vi "set output trigger source.vi"(8 "error in (no error)":errorcluster, 10 "Output trigger connector":T1=enum."3", 11 "DAQOrcaFlash in":refnum<class "DAQOrcaFlash.lvclass">) -> (0 "error out":errorcluster, 3 "DAQOrcaFlash out":refnum<class "DAQOrcaFlash.lvclass">)   [LabVIEW 2012, in "DAQOrcaFlash.lvclass"]
uses:
  DAQOrcaFlash.lvclass
  connector.ctl
  DAQOrcaFlash.lvclass/DAQOrcaFlash.ctl
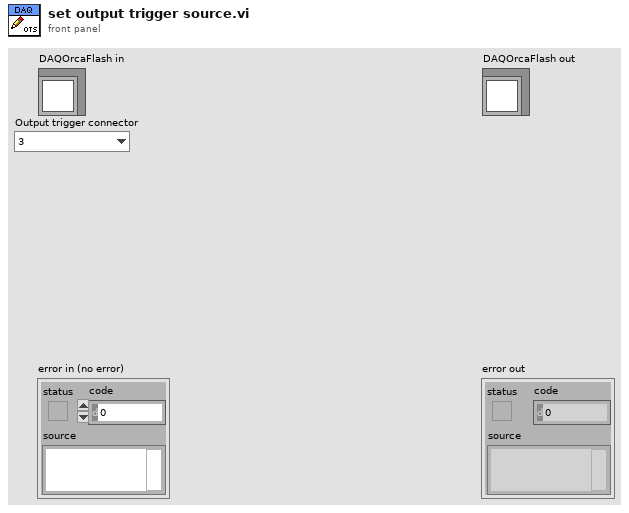
[diagram p1: front panel]
types:
  T1 = typedef "DAQOrcaFlash.lvclass/connector.ctl" = enum32{"1", "2", "3"}
  T2 = typedef "DAQOrcaFlash.lvclass/output trigger source.ctl" = sgl
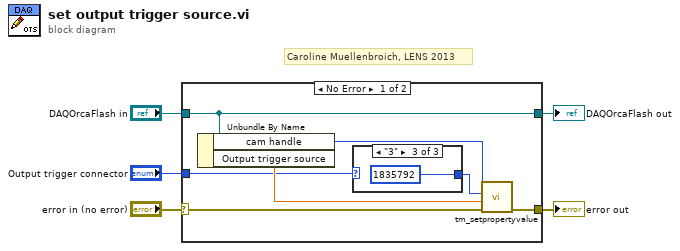
[diagram p0: block diagram]
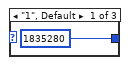
[diagram p2: hidden frame]
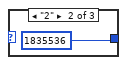
[diagram p3: hidden frame]
diagram:
  # "Caroline Muellenbroich, LENS 2013"
  n1 = case shown="No Error" "error in (no error)" {
    selector: "error in (no error)" -> [w11 w17]
    tunnel: [w10 w17] -> w4
    tunnel: [w12 w16] -> w2
    tunnel: "DAQOrcaFlash in" -> [w12 w16]
    tunnel: "Output trigger connector" -> [w6 _]
    frame No Error {
      n2 = Unbundle By Name(w12) -> ("cam handle"=w8:u32, "Output trigger source"=w9:T2)
      n3 = case shown="\"3\"" w6 {
        tunnel: [u32 1835280 ("Property ID") u32 1835536 ("Property ID") u32 1835792 ("Property ID")] -> w7
        frame "1", Default {
        }
        frame "2" {
        }
        frame "3" {
        }
      }
      n4 = call <userlib>:"tm_setpropertyvalue.vi"("error in (no error)"=w11, "Value in"=w9, "Property ID"=w7, "Handle in"=w8) -> ("error out"=w10:errorcluster)  [unwired: 6 in, 1 out]
    }
    frame Error {
    }
  }
  "error out" <- w4
  "DAQOrcaFlash out" <- w2
